vi "FindCloseTagByName.vi"(6 "offset (0)":i32, 10 "close Tag":string, 11 "string":string) -> (1 "after close tag":string, 2 "match close tag":string, 3 "before close tag":string, 4 "offset past close tag":i32)   [LabVIEW 2020]
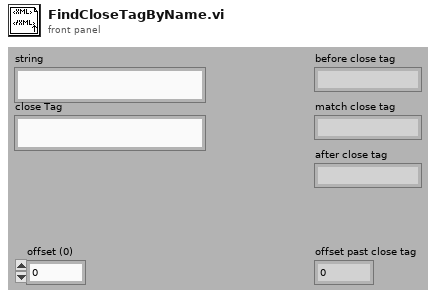
[diagram p1: front panel]
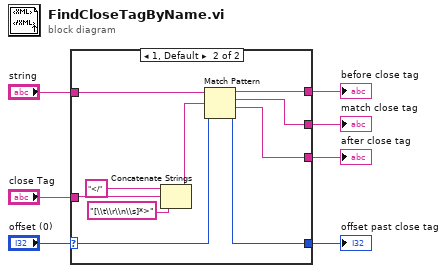
[diagram p0: block diagram]
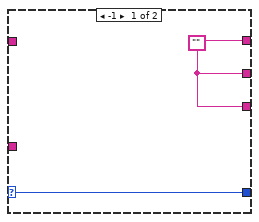
[diagram p2: hidden frame]
diagram:
  n1 = case shown="1, Default" "offset (0)" {
    selector: "offset (0)" -> [w9 w14]
    tunnel: "string" -> [_ w19]
    tunnel: "close Tag" -> [_ w12]
    tunnel: [w8 w18] -> w5
    tunnel: [w8 w17] -> w4
    tunnel: [w8 w16] -> w3
    tunnel: [w9 w15] -> w2
    frame -1 {
      w8 = ""
    }
    frame 1, Default {
      n2 = Concatenate Strings("</" ("string"), w12, "[\\t\\r\\n\\s]*>" ("regular expression")) -> (w11:string)
      n3 = Match Pattern(string=w19, regular expression=w11, offset (0)=w14) -> (before substring=w18:string, match substring=w17:string, after substring=w16:string, offset past match=w15:i32)
    }
  }
  "before close tag" <- w5
  "match close tag" <- w4
  "after close tag" <- w3
  "offset past close tag" <- w2
